vi "PDSS - Error Handling - Verify All Recipes Exist.vi"(8 "error in (no error)":errorcluster, 11 "List of Recipes":path[](array[path])=[path "c:/PDSS_observer_cbks_rcps/recipes/6563\t6563.rcp", path "c:/PDSS_observer_cbks_rcps/recipes/8542\t8542.rcp", path "c:/PDSS_observer_cbks_rcps/recipes/10830\t10830.rcp"]) -> (0 "error out":errorcluster, 1 "Recipe Not Found":path, 2 "Max cookbook Exposure [ms]":i32, 3 "No errors in cbk":bool)   [LabVIEW 2014]
doc: "Use this template to build a VI to use as a subVI."
panel:
  out "#recepies":i32
  out "Recipe Not Found":bool[](array[boolean])=[TRUE, TRUE, TRUE]
  out "All paths good":bool=TRUE
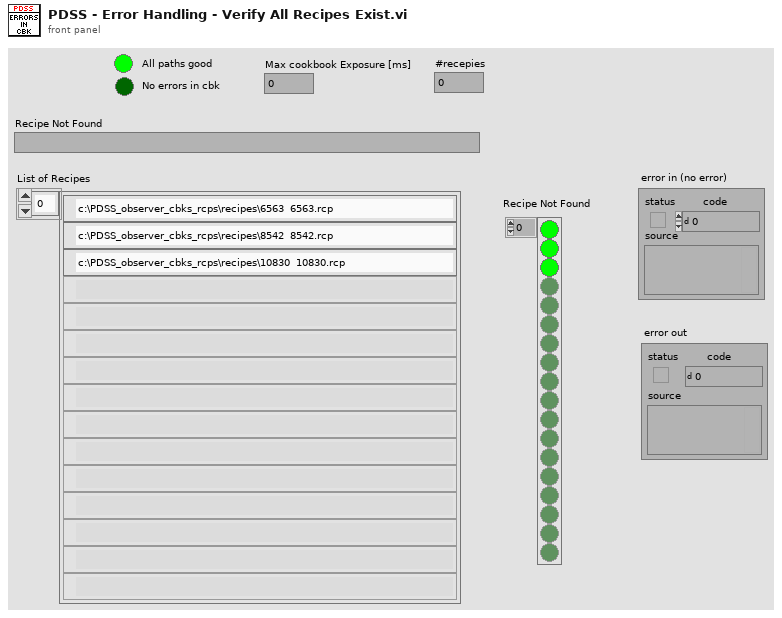
[diagram p1: front panel]
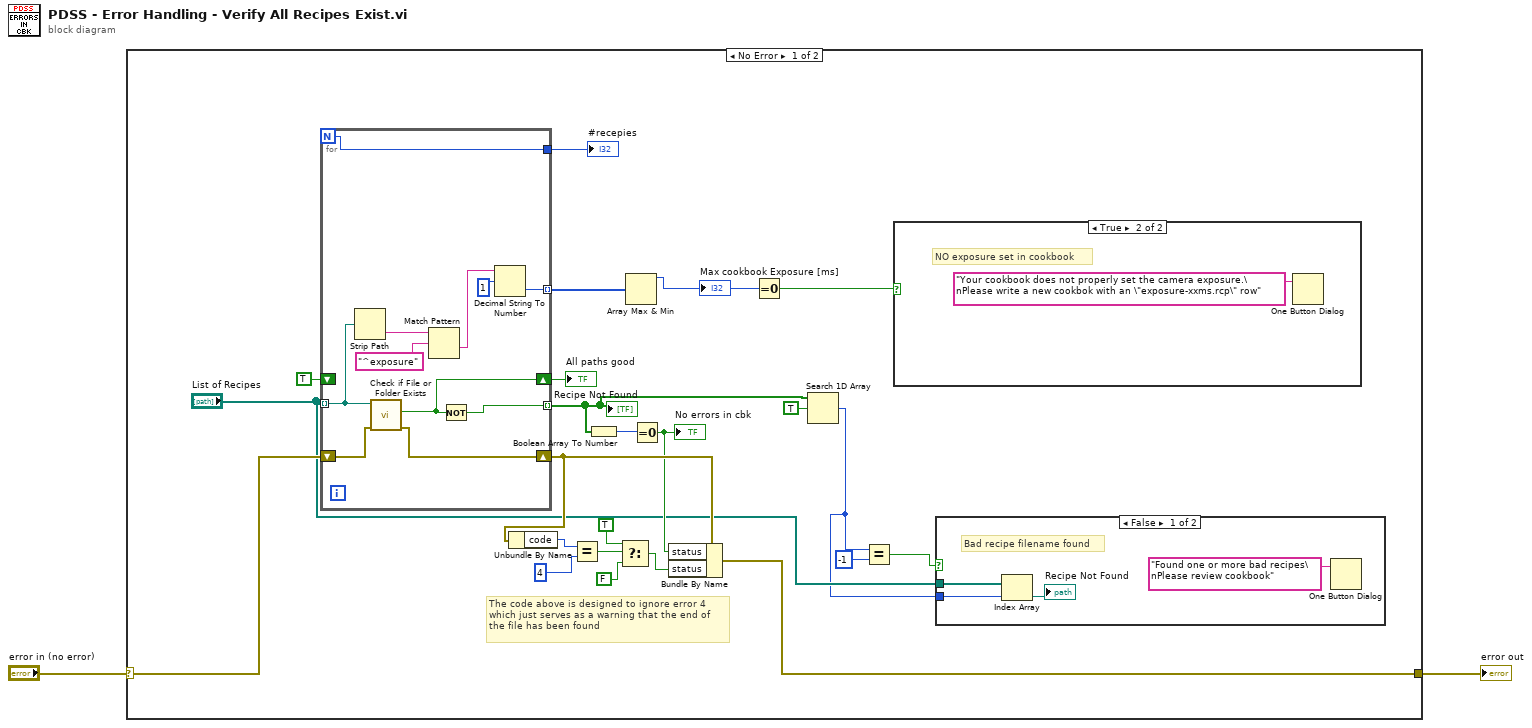
[diagram p0: block diagram]
diagram:
  n1 = case shown="No Error" "error in (no error)" {
    selector: "error in (no error)" -> [w25 w42]
    tunnel: [w21 w42] -> w1
    frame No Error {
      # "The code above is designed to ignore error 4\nwhich just serves as a warning that the end of\nthe file has been found"
      n2 = for {
        N -> [w31]
        tunnel: "List of Recipes" -> [w38] mode=indexing
        shift-right: [w40] -> w16
        shift-left: w25 -> [w41]
        shift-right: [w32] -> w23
        shift-left: TRUE ("file or folder exists?") -> [_]
        tunnel: [w39] -> w11 mode=indexing
        tunnel: [w34] -> w4 mode=indexing
        tunnel: [w31] -> w5
        n3 = Strip Path(path=w38) -> (name=w37:string)  [unwired: 1 out]
        n4 = call <vilib>:"Check if File or Folder Exists.vi"("error in (no error)"=w41, "path"=w38) -> ("error out"=w40:errorcluster, "file or folder exists?"=w32:bool)  [unwired: 7 in, 1 out]
        n5 = Match Pattern(string=w37, regular expression="^exposure") -> (after substring=w35:string)  [unwired: 1 in, 3 out]
        n6 = Not(x=w32) -> (.not. x?=w39:bool)
        n7 = Decimal String To Number(string=w35, offset=1) -> (number=w34:i32)  [unwired: 1 in, 1 out]
      }
      "All paths good" <- w23
      "Recipe Not Found" <- w11
      "#recepies" <- w5
      n8 = Unbundle By Name(w16) -> ("code"=w15:i32)
      n9 = Equal?(x=w15, y=4) -> (x = y?=w19:bool)
      n10 = Boolean Array To Number(Boolean array=w11) -> (number=w22:u32)
      n11 = Select(t=TRUE, s=w19, f=FALSE) -> (s? t:f=w14:bool)
      n12 = Array Max & Min(array=w4) -> (max value=w3:i32)  [unwired: 3 out]
      "Max cookbook Exposure [ms]" <- w3
      n13 = Equal To 0?(x=w22) -> (x = 0?=w13:bool)
      "No errors in cbk" <- w13
      n14 = Bundle By Name(cluster=w16, "status"=w13, "status"=w14) -> (w21:errorcluster)
      n15 = Equal To 0?(x=w3) -> (x = 0?=w12:bool)
      n16 = Search 1D Array(1D array=w11, element=TRUE) -> (index of element=w6:i32)  [unwired: 1 in]
      n17 = Equal?(x=w6, y=-1) -> (x = y?=w8:bool)
      n18 = case shown="True" w12 {
        frame False {
        }
        frame True {
          # "NO exposure set in cookbook"
          n19 = One Button Dialog(message="Your cookbook does not properly set the camera exposure.\nPlease write a new cookbok with an \"exposure-xxms.rcp\" row") -> ()  [unwired: 1 in, 1 out]
        }
      }
      n20 = case shown="False" w8 {
        tunnel: "List of Recipes" -> [w28 _]
        tunnel: w6 -> [w27 _]
        frame False {
          # "Bad recipe filename found"
          n21 = Index Array(array=w28, index=w27) -> (element=→"Recipe Not Found":path)
          n22 = One Button Dialog(message="Found one or more bad recipes\nPlease review cookbook") -> ()  [unwired: 1 in, 1 out]
        }
        frame True {
          # "All recipes are good"
        }
      }
    }
    frame Error {
    }
  }
  "error out" <- w1
